vi "GT Set Var Value.vi"(6 "count":i16, 7 "pValue":dbl, 8 "error in (no error)":errorcluster caption="错误输入（无错误）", 9 "pVarInfo":T1, 10 "page":i16, 11 "cardNum":i16) -> (0 "error out":errorcluster caption="错误输出", 1 "pVarInfo out":T1, 3 "function return":i16, 5 "pValue out":dbl)   [LabVIEW 2020, in "gts.lvlib"]
doc: "GT_API GT_SetVarValue(short cardNum,short page,TVarInfo *pVarInfo,double *pValue,short count=1);"
uses:
  gts.lvlib
  dll/32bit/multi_card/gts.dll
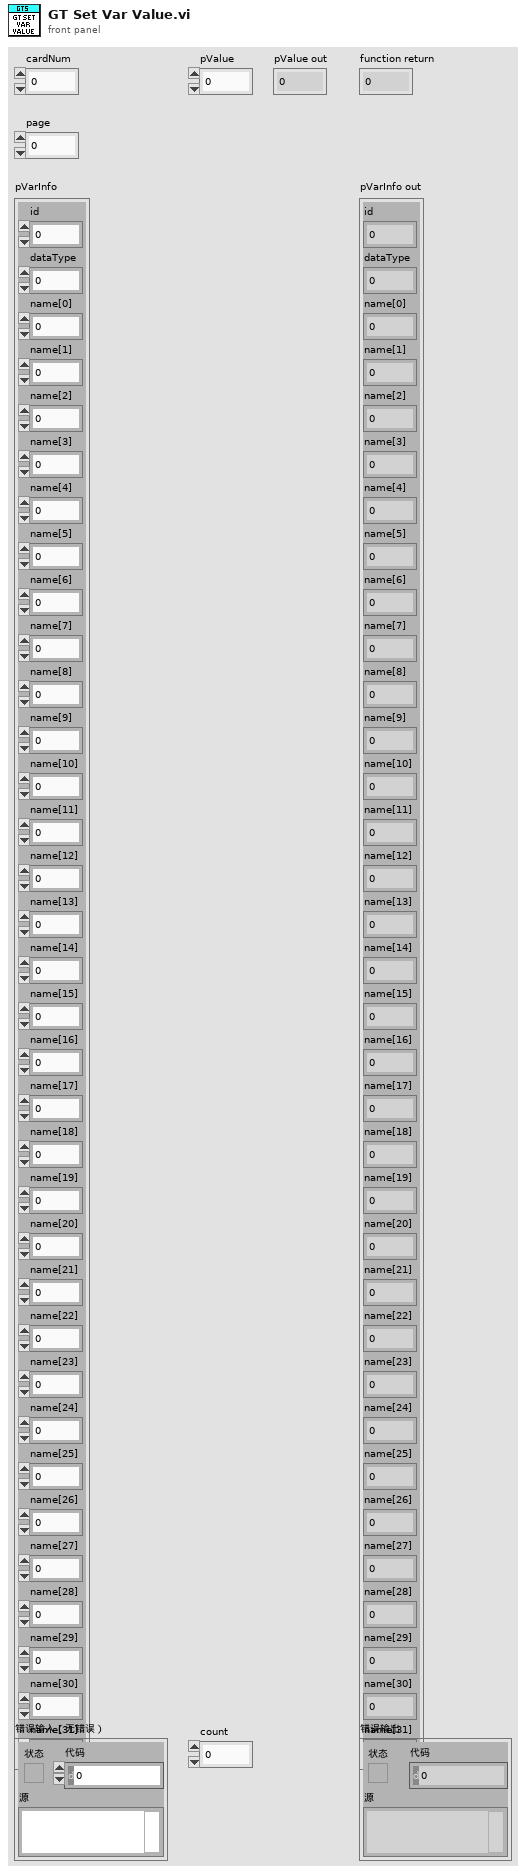
[diagram p1: front panel]
types:
  T1 = cluster{"id":i16, "dataType":i16, "name[0]":i8, "name[1]":i8, "name[2]":i8, "name[3]":i8, "name[4]":i8, "name[5]":i8, "name[6]":i8, "name[7]":i8, "name[8]":i8, "name[9]":i8, "name[10]":i8, "name[11]":i8, "name[12]":i8, "name[13]":i8, "name[14]":i8, "name[15]":i8, "name[16]":i8, "name[17]":i8, "name[18]":i8, "name[19]":i8, "name[20]":i8, "name[21]":i8, "name[22]":i8, "name[23]":i8, "name[24]":i8, "name[25]":i8, "name[26]":i8, "name[27]":i8, "name[28]":i8, "name[29]":i8, "name[30]":i8, "name[31]":i8}
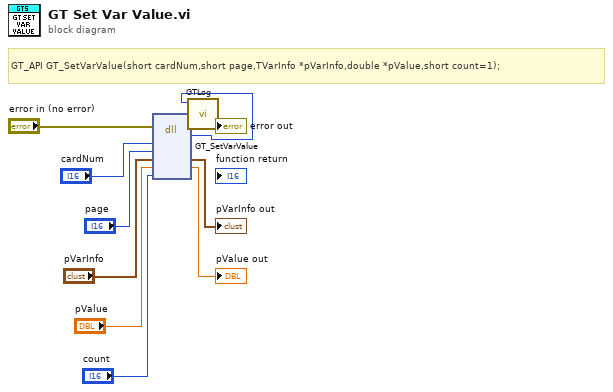
[diagram p0: block diagram]
diagram:
  # "GT_API GT_SetVarValue(short cardNum,short page,TVarInfo *pVarInfo,double *pValue,short count=1);"
  n1 = dll-call lib="C:/1228/dll/32bit/multi_card/gts.dll" fn="GT_SetVarValue"(error in="error in (no error)", "cardNum"="cardNum", "page"="page", "pVarInfo"="pVarInfo", "pValue"="pValue", "count"="count") -> (error out=w3:errorcluster, w1:i16, "pVarInfo"=→"pVarInfo out":T1, "pValue"=→"pValue out":dbl)  [unwired: 5 in, 1 out]
  n2 = call "GTLog.vi"("error in (no error)"=w3, "Numeric"=w1) -> ("error out"=→"error out":errorcluster)  [unwired: 9 in]
